vi "ConvertBetweenXYandPixel.vi"(8 "XYtoPixels":bool=TRUE, 9 "PointToConvert":cluster{sgl, sgl}, 10 "HomeXY(pixels)":cluster{dbl, dbl}, 11 "Pixel/mm":dbl format="%#_13g") -> (3 "Point":cluster{sgl, sgl})   [LabVIEW 2017]
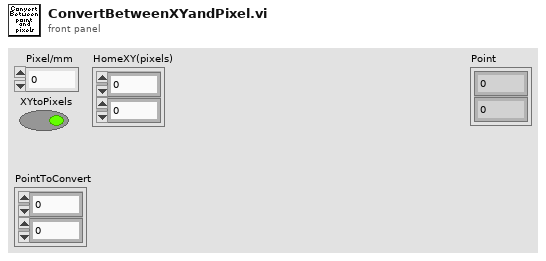
[diagram p1: front panel]
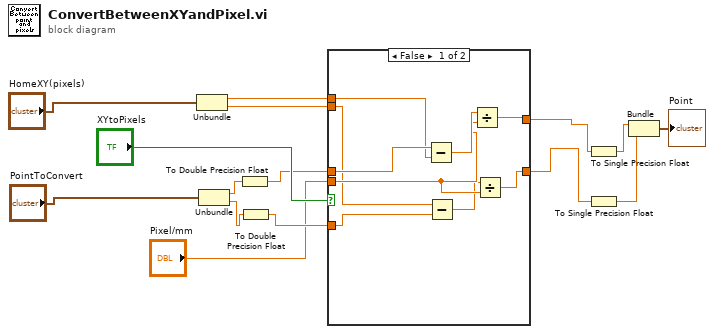
[diagram p0: block diagram]
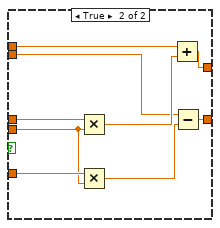
[diagram p2: hidden frame]
diagram:
  n1 = Unbundle("HomeXY(pixels)") -> (w13:dbl, w12:dbl)
  n2 = Unbundle("PointToConvert") -> (w4:sgl, w5:sgl)
  n3 = To Double Precision Float(number=w4) -> (double precision float=w3:dbl)
  n4 = To Double Precision Float(number=w5) -> (double precision float=w2:dbl)
  n5 = case shown="False" "XYtoPixels" {
    tunnel: w3 -> [w24 w33]
    tunnel: w2 -> [w16 w32]
    tunnel: "Pixel/mm" -> [w21 w25]
    tunnel: w13 -> [w23 w31]
    tunnel: w12 -> [w17 w29]
    tunnel: [w19 w27] -> w9
    tunnel: [w18 w26] -> w8
    frame False {
      n6 = Subtract(x=w24, y=w23) -> (x-y=w22:dbl)
      n7 = Subtract(x=w17, y=w16) -> (x-y=w20:dbl)
      n8 = Divide(x=w22, y=w21) -> (x/y=w19:dbl)
      n9 = Divide(x=w20, y=w21) -> (x/y=w18:dbl)
    }
    frame True {
      n10 = Multiply(x=w33, y=w25) -> (x*y=w30:dbl)
      n11 = Multiply(x=w32, y=w25) -> (x*y=w28:dbl)
      n12 = Add(x=w31, y=w30) -> (x+y=w27:dbl)
      n13 = Subtract(x=w29, y=w28) -> (x-y=w26:dbl)
    }
  }
  n14 = To Single Precision Float(number=w9) -> (single precision float=w7:sgl)
  n15 = To Single Precision Float(number=w8) -> (single precision float=w6:sgl)
  n16 = Bundle(w7, w6) -> (→"Point":cluster{sgl, sgl})  [unwired: 1 in]
